vi "Build Custom Device XML Extra Page Sections String.vi"(7 "Pages In":refnum<k20>, 8 "error in":errorcluster, 9 "Document In":refnum<k20>, 10 "Plugin Name":string, 11 "Pages Properties":T1[](array[typedef])) -> (0 "error out":errorcluster, 1 "Document Out":refnum<k20>)   [LabVIEW 2026, in "NIVS_CDEW_MetaDataObj.lvclass"]
uses:
  NIVS_CDEW_MetaDataObj.lvclass
  Types/Page Properties.ctl
  Types/Page Types.ctl
  NIVS_CDEW_MetaDataObj.lvclass/NIVS_CDEW_MetaDataObj.ctl
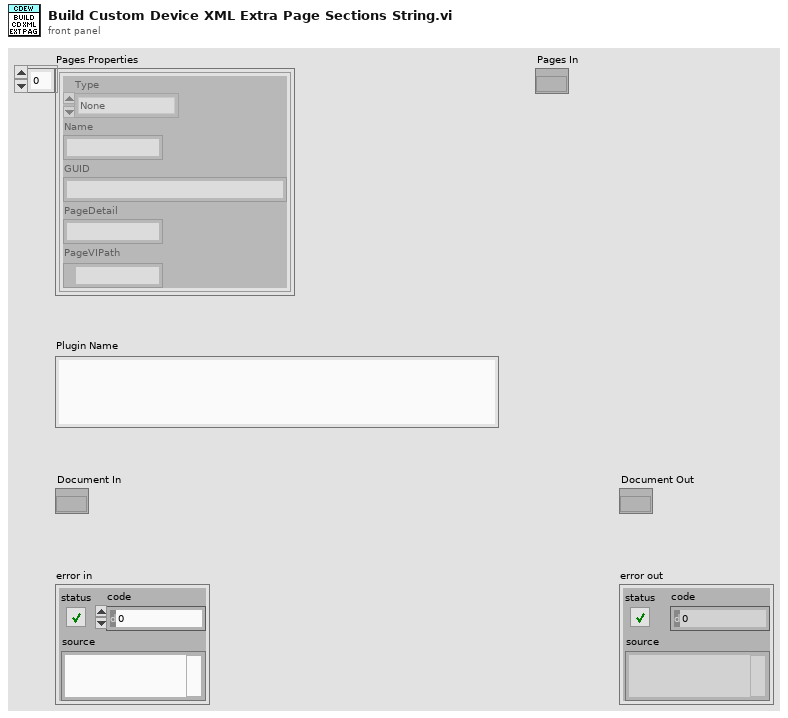
[diagram p1: front panel]
types:
  T1 = typedef "NIVS_CDEW_MetaDataObj.lvclass/Page Properties.ctl" = cluster{"Type":T2, "Name":string, "GUID":string, "PageDetail":string, "PageVIPath":path}
  T2 = typedef "NIVS_CDEW_MetaDataObj.lvclass/Page Types.ctl" = enum16{"None", "CustomDevice", "Channel", "Waveform", "Section", "DynamicChannel", "DynamicWaveform", "DynamicSection"}
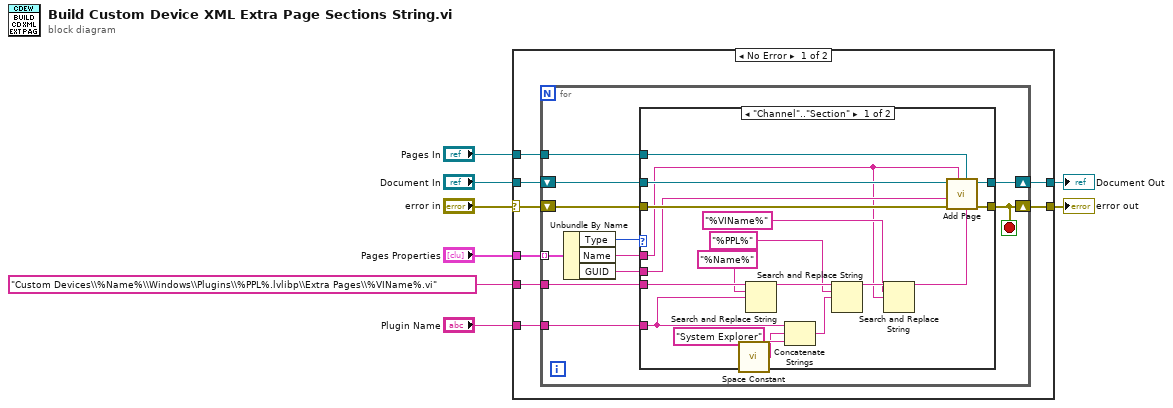
[diagram p0: block diagram]
diagram:
  n1 = case shown="No Error" "error in" {
    selector: "error in" -> [w13 w49]
    tunnel: "Pages Properties" -> [w16 _]
    tunnel: "Plugin Name" -> [w15 _]
    tunnel: [w14 w49] -> w6
    tunnel: "Custom Devices\\%Name%\\Windows\\Plugins\\%PPL%.lvlibp\\Extra Pages\\%VIName%.vi" -> [w12 _]
    tunnel: "Pages In" -> [w11 _]
    tunnel: "Document In" -> [w10 w48]
    tunnel: [w9 w48] -> w1
    frame No Error {
      n2 = for {
        tunnel: w16 -> [w27] mode=indexing
        tunnel: w15 -> [w23]
        shift-right: [w21] -> w14
        shift-left: w13 -> [w22]
        tunnel: w12 -> [w20]
        tunnel: w11 -> [w19]
        shift-right: [w17] -> w9
        shift-left: w10 -> [w18]
        stop <- w21 stop-if-true
        n3 = Unbundle By Name(w27) -> ("Type"=w26:T2, "Name"=w25:string, "GUID"=w24:string)
        n4 = case shown="\"Channel\"..\"Section\"" w26 {
          tunnel: w25 -> [w29 _]
          tunnel: w24 -> [w43 _]
          tunnel: w23 -> [w30 _]
          tunnel: [w45 w47] -> w21
          tunnel: w22 -> [w44 w47]
          tunnel: w20 -> [w37 _]
          tunnel: w19 -> [w40 _]
          tunnel: w18 -> [w39 w46]
          tunnel: [w38 w46] -> w17
          frame "Channel".."Section" {
            n5 = call <vilib>:"Space Constant.vi"() -> ("String"=w41:string)
            n6 = Search and Replace String(input string=w37, search string="%Name%", replace string=w30) -> (result string=w35:string)  [unwired: 5 in, 3 out]
            n7 = Concatenate Strings(w30, w41, "System Explorer" ("string")) -> (w34:string)
            n8 = Search and Replace String(input string=w35, search string="%PPL%", replace string=w34) -> (result string=w32:string)  [unwired: 5 in, 3 out]
            n9 = Search and Replace String(input string=w32, search string="%VIName%", replace string=w29) -> (result string=w28:string)  [unwired: 5 in, 3 out]
            n10 = call "Add Page.vi"("Path"=w28, "Pages In"=w40, "Name"=w29, "error in"=w44, "GUID"=w43, "Document In"=w39) -> ("error out"=w45:errorcluster, "Document out"=w38:refnum<k20>)  [unwired: 4 in]
          }
          frame "None", "CustomDevice", "DynamicChannel".."DynamicSection" {
          }
        }
      }
    }
    frame Error {
    }
  }
  "error out" <- w6
  "Document Out" <- w1
